vi "checkUDP.vi"(8 "error in (no error)":errorcluster, 11 "Mockbus in":refnum<class "Mockbus.lvclass">) -> (0 "error out":errorcluster, 3 "Mockbus out":refnum<class "Mockbus.lvclass">)   [LabVIEW 2015, in "Mockbus.lvclass"]
uses:
  Mockbus.lvclass
  Typedefs/Frame.ctl
  Typedefs/RTTypeDefs.lvlib
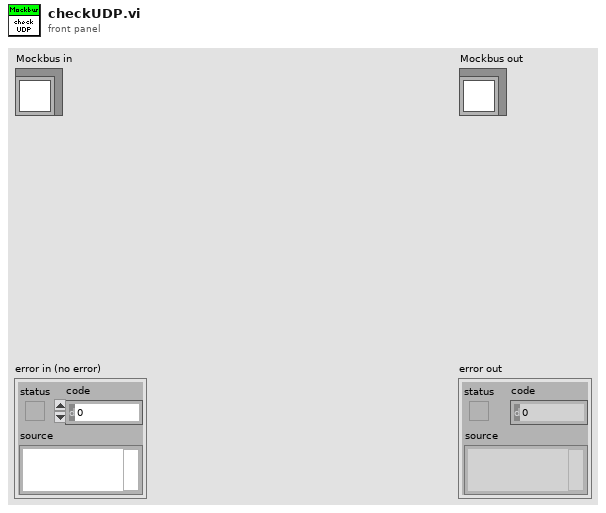
[diagram p1: front panel]
types:
  T1 = typedef "RTTypeDefs.lvlib/UDPCommand.ctl" = cluster{"Command":string, "Data":u8[]}
  T2 = typedef "RTTypeDefs.lvlib/Frame.ctl" = cluster{"Data":u8[]}
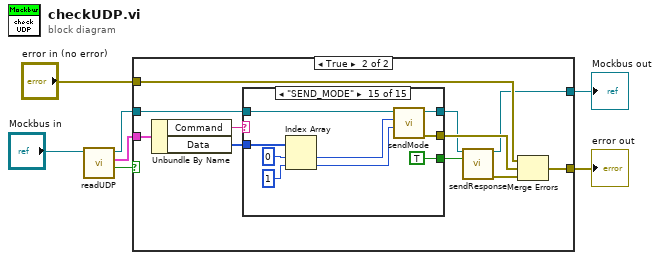
[diagram p0: block diagram]
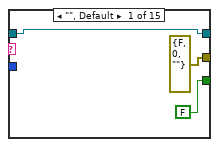
[diagram p3: hidden frame]
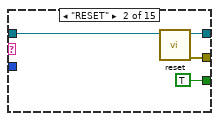
[diagram p4: hidden frame]
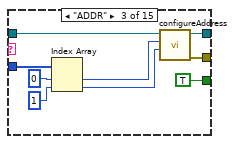
[diagram p5: hidden frame]
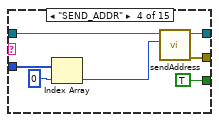
[diagram p6: hidden frame]
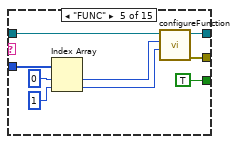
[diagram p7: hidden frame]
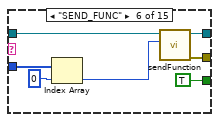
[diagram p8: hidden frame]
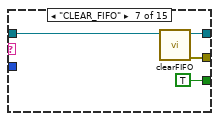
[diagram p9: hidden frame]
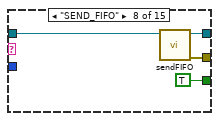
[diagram p10: hidden frame]
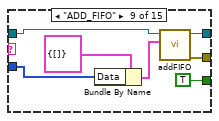
[diagram p11: hidden frame]
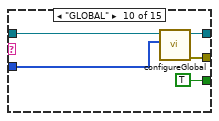
[diagram p12: hidden frame]
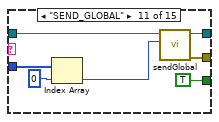
[diagram p13: hidden frame]
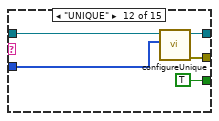
[diagram p14: hidden frame]
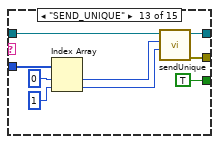
[diagram p15: hidden frame]
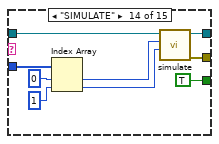
[diagram p16: hidden frame]
diagram:
  n1 = call "readUDP.vi"("Mockbus in"="Mockbus in") -> ("CommandAvailable"=w4:bool, "UDP Command"=w6:T1, "Mockbus out"=w5:refnum<class "Mockbus.lvclass">)  [unwired: 7 in, 1 out]
  n2 = case shown="True" w4 {
    tunnel: w6 -> [_ w20]
    tunnel: w5 -> [w9 w18]
    tunnel: "error in (no error)" -> [w8 w12]
    tunnel: [w8 w11] -> w2
    tunnel: [w9 w10] -> w1
    frame False {
    }
    frame True {
      n3 = Unbundle By Name(w20) -> ("Command"=w19:string, "Data"=w16:u8[])
      n4 = case shown="\"SEND_MODE\"" w19 {
        tunnel: w18 -> [w22 w27 w36 w43 w52 w59 w63 w67 w72 w79 w86 w90 w95 w104 w113]
        tunnel: [w22 w26 w29 w38 w45 w54 w62 w66 w70 w78 w85 w89 w94 w103 w112] -> w14
        tunnel: [errorcluster {"status"=FALSE, "code"=0, "source"=""} ("error out") w25 w30 w39 w46 w55 w61 w65 w71 w77 w84 w88 w93 w102 w111] -> w17
        tunnel: w16 -> [_ _ w35 w42 w51 w58 _ _ w69 w76 w82 w91 w100 w109 w118]
        tunnel: [FALSE TRUE TRUE TRUE TRUE TRUE TRUE TRUE TRUE TRUE TRUE TRUE TRUE TRUE TRUE] -> w15
        frame "", Default {
        }
        frame "RESET" {
          n5 = call "reset.vi"("Mockbus in"=w27) -> ("error out"=w25:errorcluster, "Mockbus out"=w26:refnum<class "Mockbus.lvclass">)  [unwired: 9 in]
        }
        frame "ADDR" {
          n6 = Index Array(array=w35, index #1=0 ("index"), index #2=1 ("index")) -> (element #1=w32:u8, element #2=w31:u8)
          n7 = call "configureAddress.vi"("Config"=w31, "Address"=w32, "Mockbus in"=w36) -> ("error out"=w30:errorcluster, "Mockbus out"=w29:refnum<class "Mockbus.lvclass">)  [unwired: 7 in]
        }
        frame "SEND_ADDR" {
          n8 = Index Array(array=w42, index=0) -> (element=w40:u8)
          n9 = call "sendAddress.vi"("Address"=w40, "Mockbus in"=w43) -> ("error out"=w39:errorcluster, "Mockbus out"=w38:refnum<class "Mockbus.lvclass">)  [unwired: 8 in]
        }
        frame "FUNC" {
          n10 = Index Array(array=w51, index #1=0 ("index"), index #2=1 ("index")) -> (element #1=w48:u8, element #2=w47:u8)
          n11 = call "configureFunction.vi"("Config"=w47, "Function"=w48, "Mockbus in"=w52) -> ("error out"=w46:errorcluster, "Mockbus out"=w45:refnum<class "Mockbus.lvclass">)  [unwired: 7 in]
        }
        frame "SEND_FUNC" {
          n12 = Index Array(array=w58, index=0) -> (element=w56:u8)
          n13 = call "sendFunction.vi"("Function"=w56, "Mockbus in"=w59) -> ("error out"=w55:errorcluster, "Mockbus out"=w54:refnum<class "Mockbus.lvclass">)  [unwired: 8 in]
        }
        frame "CLEAR_FIFO" {
          n14 = call "clearFIFO.vi"("Mockbus in"=w63) -> ("error out"=w61:errorcluster, "Mockbus out"=w62:refnum<class "Mockbus.lvclass">)  [unwired: 9 in]
        }
        frame "SEND_FIFO" {
          n15 = call "sendFIFO.vi"("Mockbus in"=w67) -> ("error out"=w65:errorcluster, "Mockbus out"=w66:refnum<class "Mockbus.lvclass">)  [unwired: 9 in]
        }
        frame "ADD_FIFO" {
          n16 = Bundle By Name(cluster=T2 {"Data"=[]} ("Frame"), "Data"=w69) -> (w73:T2)
          n17 = call "addFIFO.vi"("Frame"=w73, "Mockbus in"=w72) -> ("error out"=w71:errorcluster, "Mockbus out"=w70:refnum<class "Mockbus.lvclass">)  [unwired: 8 in]
        }
        frame "GLOBAL" {
          n18 = call "configureGlobal.vi"("Data"=w76, "Mockbus in"=w79) -> ("error out"=w77:errorcluster, "Mockbus out"=w78:refnum<class "Mockbus.lvclass">)  [unwired: 8 in]
        }
        frame "SEND_GLOBAL" {
          n19 = Index Array(array=w82, index=0) -> (element=w80:u8)
          n20 = call "sendGlobal.vi"("Function"=w80, "Mockbus in"=w86) -> ("error out"=w84:errorcluster, "Mockbus out"=w85:refnum<class "Mockbus.lvclass">)  [unwired: 8 in]
        }
        frame "UNIQUE" {
          n21 = call "configureUnique.vi"("Data"=w91, "Mockbus in"=w90) -> ("error out"=w88:errorcluster, "Mockbus out"=w89:refnum<class "Mockbus.lvclass">)  [unwired: 8 in]
        }
        frame "SEND_UNIQUE" {
          n22 = Index Array(array=w100, index #1=0 ("index"), index #2=1 ("index")) -> (element #1=w97:u8, element #2=w96:u8)
          n23 = call "sendUnique.vi"("Function"=w96, "Address"=w97, "Mockbus in"=w95) -> ("error out"=w93:errorcluster, "Mockbus out"=w94:refnum<class "Mockbus.lvclass">)  [unwired: 7 in]
        }
        frame "SIMULATE" {
          n24 = Index Array(array=w109, index #1=0 ("index"), index #2=1 ("index")) -> (element #1=w106:u8, element #2=w105:u8)
          n25 = call "simulate.vi"("Function"=w105, "Address"=w106, "Mockbus in"=w104) -> ("error out"=w102:errorcluster, "Mockbus out"=w103:refnum<class "Mockbus.lvclass">)  [unwired: 7 in]
        }
        frame "SEND_MODE" {
          n26 = Index Array(array=w118, index #1=0 ("index"), index #2=1 ("index")) -> (element #1=w115:u8, element #2=w114:u8)
          n27 = call "sendMode.vi"("Function"=w114, "Address"=w115, "Mockbus in"=w113) -> ("error out"=w111:errorcluster, "Mockbus out"=w112:refnum<class "Mockbus.lvclass">)  [unwired: 7 in]
        }
      }
      n28 = call "sendResponse.vi"("Mockbus in"=w14, "AllGood?"=w15) -> ("Mockbus out"=w10:refnum<class "Mockbus.lvclass">, "error out"=w13:errorcluster)  [unwired: 12 in]
      n29 = Merge Errors(w12, w17, w13) -> (w11:errorcluster)
    }
  }
  "error out" <- w2
  "Mockbus out" <- w1
